vi "p1.vi"() -> ()   [LabVIEW 2021, in "d5.lvlib"]
uses:
  d5.lvlib
  AOC/AOC.lvlib
panel:
  in  "Example":string="    [D]    \n[N] [C]    \n[Z] [M] [P]\n 1   2   3 \n\nmove 1 from 2 to 1\nmove 3 from 1 to 3\nmove 2 from 2 to 1\nmove 1 from 1 to 2"
  in  "Example":bool
  out "Answer":string
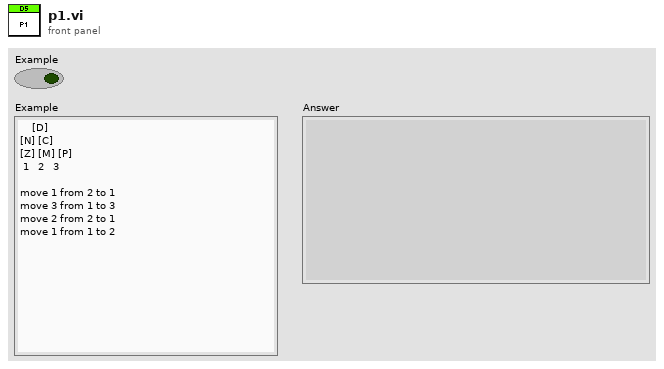
[diagram p1: front panel]
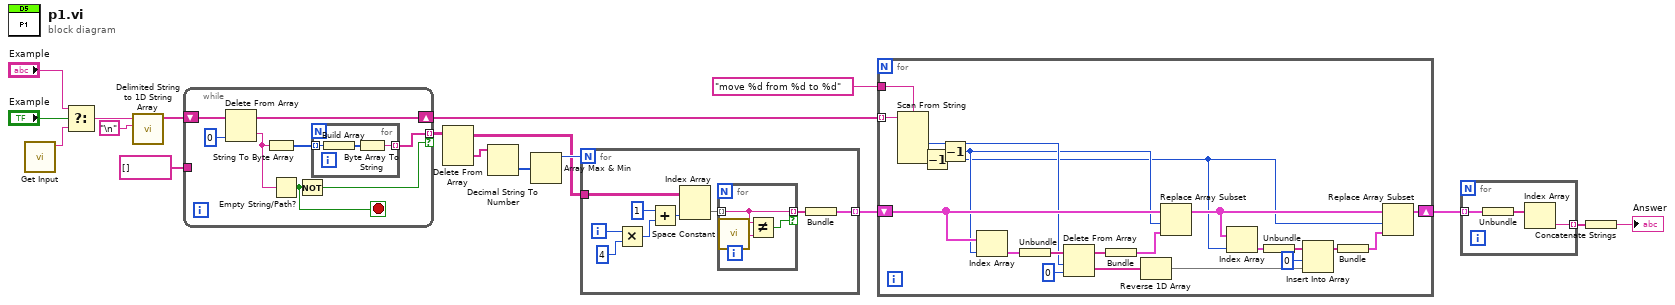
[diagram p0: block diagram]
diagram:
  n1 = call "Get Input.vi"() -> ("Input"=w18:string)  [unwired: 11 in]
  n2 = Select(t="Example", s="Example", f=w18) -> (s? t:f=w17:string)
  n3 = call <vilib>:"Delimited String to 1D String Array.vi"("delimiter"="\n", "delimited string"=w17) -> ("string array"=w13:string[])  [unwired: 9 in]
  n4 = while {
    shift-right: [w25] -> w7
    shift-left: w13 -> [w26]
    tunnel: [w19] -> w12 mode=indexing if=w23
    tunnel: string[] [] ("string array") -> [_]
    stop <- w22 stop-if-true
    n5 = Delete From Array(array=w26, index=0) -> (deleted portion=w21:string, array with subset deleted=w25:string[])  [unwired: 1 in]
    n6 = String To Byte Array(string=w21) -> (unsigned byte array=w20:u8[])
    n7 = Empty String/Path?(string/path=w21) -> (empty?=w22:bool)
    n8 = Not(x=w22) -> (.not. x?=w23:bool)
    n9 = for {
      tunnel: w20 -> [w29] mode=indexing
      tunnel: [w27] -> w19 mode=indexing
      n10 = Build Array(w29) -> (w28:u8[])
      n11 = Byte Array To String(unsigned byte array=w28) -> (string=w27:string)
    }
  }
  n12 = Delete From Array(array=w12) -> (deleted portion=w8:string[], array with subset deleted=w9:string[][])  [unwired: 3 in]
  n13 = Decimal String To Number(string=w8) -> (number=w11:i32[])  [unwired: 2 in, 1 out]
  n14 = Array Max & Min(array=w11) -> (max value=w10:i32)  [unwired: 3 out]
  n15 = for {
    N: w10 -> [_]
    tunnel: w9 -> [w38]
    tunnel: [w36] -> w6 mode=indexing
    i -> [w37]
    n16 = Multiply(x=w37, y=4) -> (x*y=w35:i32)
    n17 = Add(x=1, y=w35) -> (x+y=w33:i32)
    n18 = Index Array(array=w38, index (col)=w33) -> (element=w31:string[])  [unwired: 1 in]
    n19 = for {
      tunnel: w31 -> [w41] mode=indexing
      tunnel: [w41] -> w30 mode=indexing if=w40
      n20 = call <vilib>:"Space Constant.vi"() -> ("String"=w39:string)
      n21 = Not Equal?(x=w41, y=w39) -> (x != y?=w40:bool)
    }
    n22 = Bundle(w30) -> (w36:cluster{string[]})  [unwired: 1 in]
  }
  n23 = for {
    tunnel: w7 -> [w63] mode=indexing
    tunnel: "move %d from %d to %d" ("format string") -> [w62]
    shift-right: [w48] -> w4
    shift-left: w6 -> [w58]
    n24 = Scan From String(format string=w62, input string=w63) -> (output 1=w44:i32, output 2=w46:i32, output 3=w47:i32)  [unwired: 5 in, 3 out]
    n25 = Decrement(x=w47) -> (x-1=w42:i32)
    n26 = Decrement(x=w46) -> (x-1=w43:i32)
    n27 = Index Array(array=w58, index=w43) -> (element=w61:cluster{string[]})
    n28 = Unbundle(w61) -> (w60:string[])
    n29 = Delete From Array(array=w60, length=w44, index=0) -> (deleted portion=w55:string[], array with subset deleted=w57:string[])
    n30 = Bundle(w57) -> (w56:cluster{string[]})  [unwired: 1 in]
    n31 = Reverse 1D Array(array=w55) -> (reversed array=w53:string[])
    n32 = Replace Array Subset(array=w58, new element=w56, index=w43) -> (w49:cluster{string[]}[])
    n33 = Index Array(array=w49, index=w42) -> (element=w54:cluster{string[]})
    n34 = Unbundle(w54) -> (w52:string[])
    n35 = Insert Into Array(array=w52, index=0, new element=w53) -> (w50:string[])
    n36 = Bundle(w50) -> (w45:cluster{string[]})  [unwired: 1 in]
    n37 = Replace Array Subset(array=w49, new element=w45, index=w42) -> (w48:cluster{string[]}[])
  }
  n38 = for {
    tunnel: w4 -> [w66] mode=indexing
    tunnel: [w64] -> w3 mode=indexing
    n39 = Unbundle(w66) -> (w65:string[])
    n40 = Index Array(array=w65) -> (element=w64:string)  [unwired: 1 in]
  }
  n41 = Concatenate Strings(w3) -> (→"Answer":string)
